vi "Set Macro by Name.vi"(8 "error in (no error)":errorcluster, 9 "TriggerAction Q.lvclass":refnum<class "TriggerAction Q.lvclass">, 10 "Macro Name":string, 11 "Motions in":refnum<class "Motions.lvclass">) -> (0 "error out":errorcluster, 2 "replaced":bool, 3 "Motions out":refnum<class "Motions.lvclass">)   [LabVIEW 2016, in "Hardware.lvlib" / "Motions.lvlib" / "Motions.lvclass"]
uses:
  <userlib>/Common Components/Hardware/Abstract System/Motions/Motions/Motions.lvclass
  <userlib>/Common Components/TriggerAction Q/TriggerAction Q/TriggerAction Q.lvclass
  <userlib>/Common Components/Hardware/Abstract System/Motions/Motions/Motions.lvclass/Motions.ctl
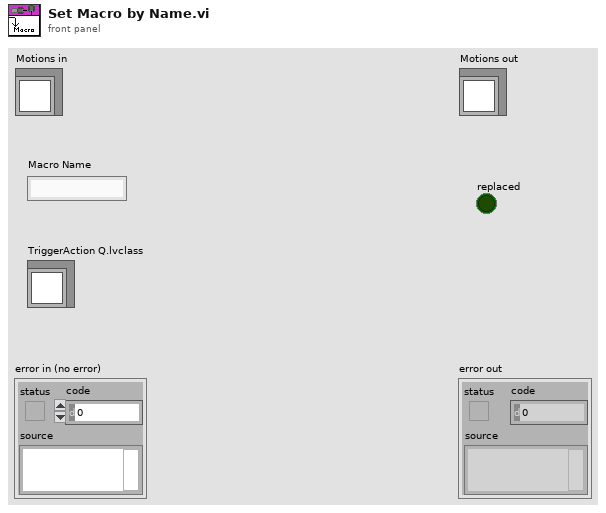
[diagram p1: front panel]
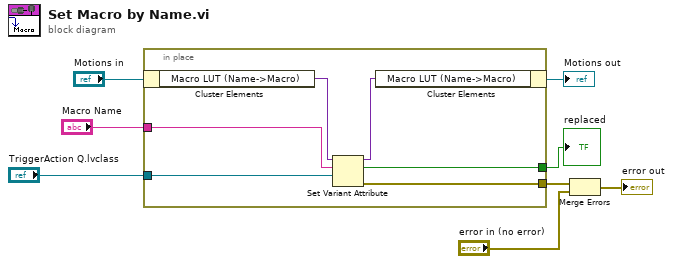
[diagram p0: block diagram]
diagram:
  n1 = in-place {
    in-place-border: "Macro Name" -> [w12]
    in-place-border: "TriggerAction Q.lvclass" -> [w11]
    in-place-border: [w10] -> w3
    in-place-border: [w9] -> w1
    n2 = in-place-cluster #1("Motions in") -> ("Macro LUT (Name->Macro)"=w14:variant)
    n3 = Set Variant Attribute(Variant=w14, name=w12, value=w11) -> (Variant out=w13:variant, replaced=w9:bool, error out=w10:errorcluster)  [unwired: 1 in]
    n4 = in-place-cluster #1("Macro LUT (Name->Macro)"=w13) -> (→"Motions out":refnum<class "Motions.lvclass">)
  }
  "replaced" <- w1
  n5 = Merge Errors(w3, "error in (no error)") -> (→"error out":errorcluster)
